vi "Kinect(SubVI).vi"(11 "refnum name":string="RobotDrive") -> ()   [LabVIEW 2011]
uses:
  <vilib>/addons/Kinect/Skeleton Vertex Index.ctl
  <vilib>/addons/Kinect/SkeletonVertexTrackState.ctl
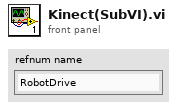
[diagram p1: front panel]
types:
  T1 = typedef "SkeletonVertexTrackState.ctl" = enum32{"NotTracked", "Inferred", "Tracked"}
  T2 = typedef "Skeleton Vertex Index.ctl" = i32
  T3 = typedef "WPI_RobotDriveDevRef.ctl" = cluster{"DevStatus":errorcluster, "Motors[]":T4[], "Square Inputs":bool, "Max Output":dbl, "Isochronous":bool}
  T4 = typedef "WPI_MotorControlDeviceRef.ctl" = cluster{"DeviceStatus":errorcluster, "Type":enum16{"PWM", "CAN"}, "PWM":cluster{"Digital Module":T5, "PWM Channel":T6, "DeadBand":T7}, "CAN":cluster{"Device Number":u8, "Control Mode":T8, "Semaphore":T9, "Max Vout":dbl}, "Invert":bool, "TransformRef":T10, "InvTransformRef":T10}
  T5 = typedef "FPGA_TypedefDigitalModule.ctl" = enum16{"Digital Module 1", "Digital Module 2"}
  T6 = typedef "FPGA_DIOPWMChannel.ctl" = enum8{"PWM 1", "PWM 2", "PWM 3", "PWM 4", "PWM 5", "PWM 6", "PWM 7", "PWM 8", "PWM 9", "PWM 10", "Invalid"}
  T7 = typedef "WPI_PWMDeadband.ctl" = cluster{"Name":string, "maxPositivePwm":i32, "minPositivePwm":i32, "centerPwm":i32, "maxNegativePwm":i32, "minNegativePwm":i32, "angularRange":u16}
  T8 = typedef "WPI_CANJaguar_ControlMode.ctl" = enum8{"Percent VBus", "Current", "Speed", "Position", "Voltage"}
  T9 = typedef "Semaphore RefNum" = refnum<k1>
  T10 = typedef "WPI_PWMTransform_ConPane.ctl" = refnum<vi>
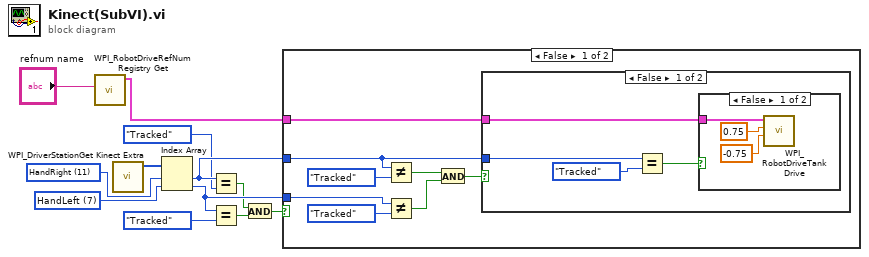
[diagram p0: block diagram]
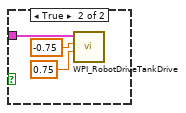
[diagram p2: hidden frame]
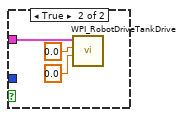
[diagram p3: hidden frame]
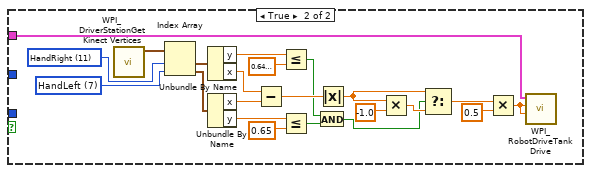
[diagram p4: hidden frame]
diagram:
  w4 = T2 7 items=["HipCenter", "Spine", "ShoulderCenter", "Head", "ShoulderLeft", "ElbowLeft", "WristLeft", "HandLeft", "ShoulderRight", "ElbowRight", "WristRight", "HandRight", "HipLeft", "KneeLeft", "AnkleLeft", "FootLeft", "HipRight", "KneeRight", "AnkleRight", "FootRight"] ("Skeleton Joints")
  w3 = T2 11 items=["HipCenter", "Spine", "ShoulderCenter", "Head", "ShoulderLeft", "ElbowLeft", "WristLeft", "HandLeft", "ShoulderRight", "ElbowRight", "WristRight", "HandRight", "HipLeft", "KneeLeft", "AnkleLeft", "FootLeft", "HipRight", "KneeRight", "AnkleRight", "FootRight"] ("Skeleton Joints")
  n1 = call <vilib>:"WPI_RobotDriveRefNum Registry Get.vi"("refnum name"="refnum name") -> ("RobotDriveDevRef"=w12:T3)  [unwired: 9 in, 1 out]
  n2 = call <vilib>:"WPI_DriverStationGet Kinect Extra.vi"() -> ("Skeleton Tracking State"=w2:T1[])  [unwired: 7 in, 4 out]
  n3 = Index Array(array=w2, index #1=w3, index #2=w4) -> (element #1=w11:T1, element #2=w10:T1)
  n4 = Equal?(x=w11, y=SkeletonVertexTrackState."Tracked") -> (x = y?=w8:bool)
  n5 = Equal?(x=w10, y=SkeletonVertexTrackState."Tracked") -> (x = y?=w7:bool)
  n6 = And(x=w8, y=w7) -> (x .and. y?=w9:bool)
  n7 = case shown="False" w9 {
    tunnel: w12 -> [w13 w49]
    tunnel: w10 -> [w20 _]
    tunnel: w11 -> [w17 _]
    frame False {
      n8 = Not Equal?(x=w17, y=SkeletonVertexTrackState."Tracked") -> (x != y?=w16:bool)
      n9 = Not Equal?(x=w20, y=SkeletonVertexTrackState."Tracked") -> (x != y?=w15:bool)
      n10 = And(x=w16, y=w15) -> (x .and. y?=w14:bool)
      n11 = case shown="False" w14 {
        tunnel: w17 -> [w24 _]
        tunnel: w13 -> [w21 w33]
        frame False {
          n12 = Equal?(x=w24, y=SkeletonVertexTrackState."Tracked") -> (x = y?=w22:bool)
          n13 = case shown="False" w22 {
            tunnel: w21 -> [w25 w28]
            frame False {
              n14 = call <vilib>:"WPI_RobotDriveTankDrive.vi"("Right axis value"=-0.75, "Left axis value"=0.75, "RobotDriveDevRef"=w25) -> ()  [unwired: 7 in, 2 out]
            }
            frame True {
              n15 = call <vilib>:"WPI_RobotDriveTankDrive.vi"("Right axis value"=0.75, "Left axis value"=-0.75, "RobotDriveDevRef"=w28) -> ()  [unwired: 7 in, 2 out]
            }
          }
        }
        frame True {
          n16 = call <vilib>:"WPI_RobotDriveTankDrive.vi"("Right axis value"=0.0, "Left axis value"=0.0, "RobotDriveDevRef"=w33) -> ()  [unwired: 7 in, 2 out]
        }
      }
    }
    frame True {
      w53 = T2 7 items=["HipCenter", "Spine", "ShoulderCenter", "Head", "ShoulderLeft", "ElbowLeft", "WristLeft", "HandLeft", "ShoulderRight", "ElbowRight", "WristRight", "HandRight", "HipLeft", "KneeLeft", "AnkleLeft", "FootLeft", "HipRight", "KneeRight", "AnkleRight", "FootRight"] ("Skeleton Joints")
      w54 = T2 11 items=["HipCenter", "Spine", "ShoulderCenter", "Head", "ShoulderLeft", "ElbowLeft", "WristLeft", "HandLeft", "ShoulderRight", "ElbowRight", "WristRight", "HandRight", "HipLeft", "KneeLeft", "AnkleLeft", "FootLeft", "HipRight", "KneeRight", "AnkleRight", "FootRight"] ("Skeleton Joints")
      n17 = call <vilib>:"WPI_DriverStationGet Kinect Vertices.vi"() -> ("Skeleton Vertices"=w55:cluster{"x":sgl, "y":sgl, "z":sgl}[])  [unwired: 10 in, 1 out]
      n18 = Index Array(array=w55, index #1=w54, index #2=w53) -> (element #1=w52:cluster{"x":sgl, "y":sgl, "z":sgl}, element #2=w51:cluster{"x":sgl, "y":sgl, "z":sgl})
      n19 = Unbundle By Name(w52) -> ("y"=w35:sgl, "x"=w46:sgl)
      n20 = Unbundle By Name(w51) -> ("x"=w45:sgl, "y"=w34:sgl)
      n21 = Subtract(x=w46, y=w45) -> (x-y=w50:sgl)
      n22 = Less Or Equal?(x=w35, y=sgl 0.65) -> (x <= y?=w38:bool)
      n23 = Less Or Equal?(x=w34, y=0.65) -> (x <= y?=w39:bool)
      n24 = And(x=w38, y=w39) -> (x .and. y?=w37:bool)
      n25 = Absolute Value(x=w50) -> (abs(x)=w41:sgl)
      n26 = Multiply(x=w41, y=-1.0) -> (x*y=w42:dbl)
      n27 = Select(t=w41, s=w37, f=w42) -> (s? t:f=w44:dbl)
      n28 = Multiply(x=w44, y=sgl 0.5) -> (x*y=w48:dbl)
      n29 = call <vilib>:"WPI_RobotDriveTankDrive.vi"("Right axis value"=w48, "Left axis value"=w48, "RobotDriveDevRef"=w49) -> ()  [unwired: 7 in, 2 out]
    }
  }
